vi "getXMLCameraPlacement.vi"(9 "usb/watec":bool, 11 "path to XML document":path=path "C:/BeamPointing/trunk/Beam Pointing v22 Library/xml Settings/ConfigFile.xml") -> (0 "error out":errorcluster, 1 "parse errors":string, 2 "Default devices":string[](array[string]), 3 "Cameras names/#":T1(array[cluster]), 5 "Default Cameras Names":string[](array[string]))   [LabVIEW 2013]
uses:
  <vilib>/xml/Load XML File.vi
  <vilib>/xml/NI_XML.lvlib
  <resource>/objmgr/DOMUserDefRef.rc
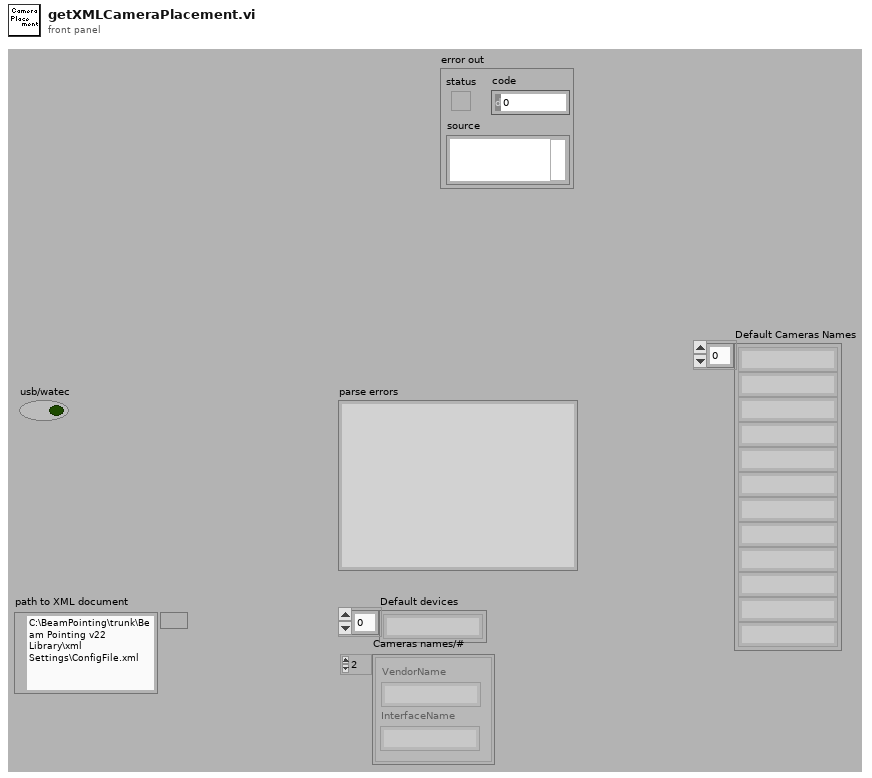
[diagram p1: front panel]
types:
  T1 = cluster{"VendorName":string, "InterfaceName":string}[]
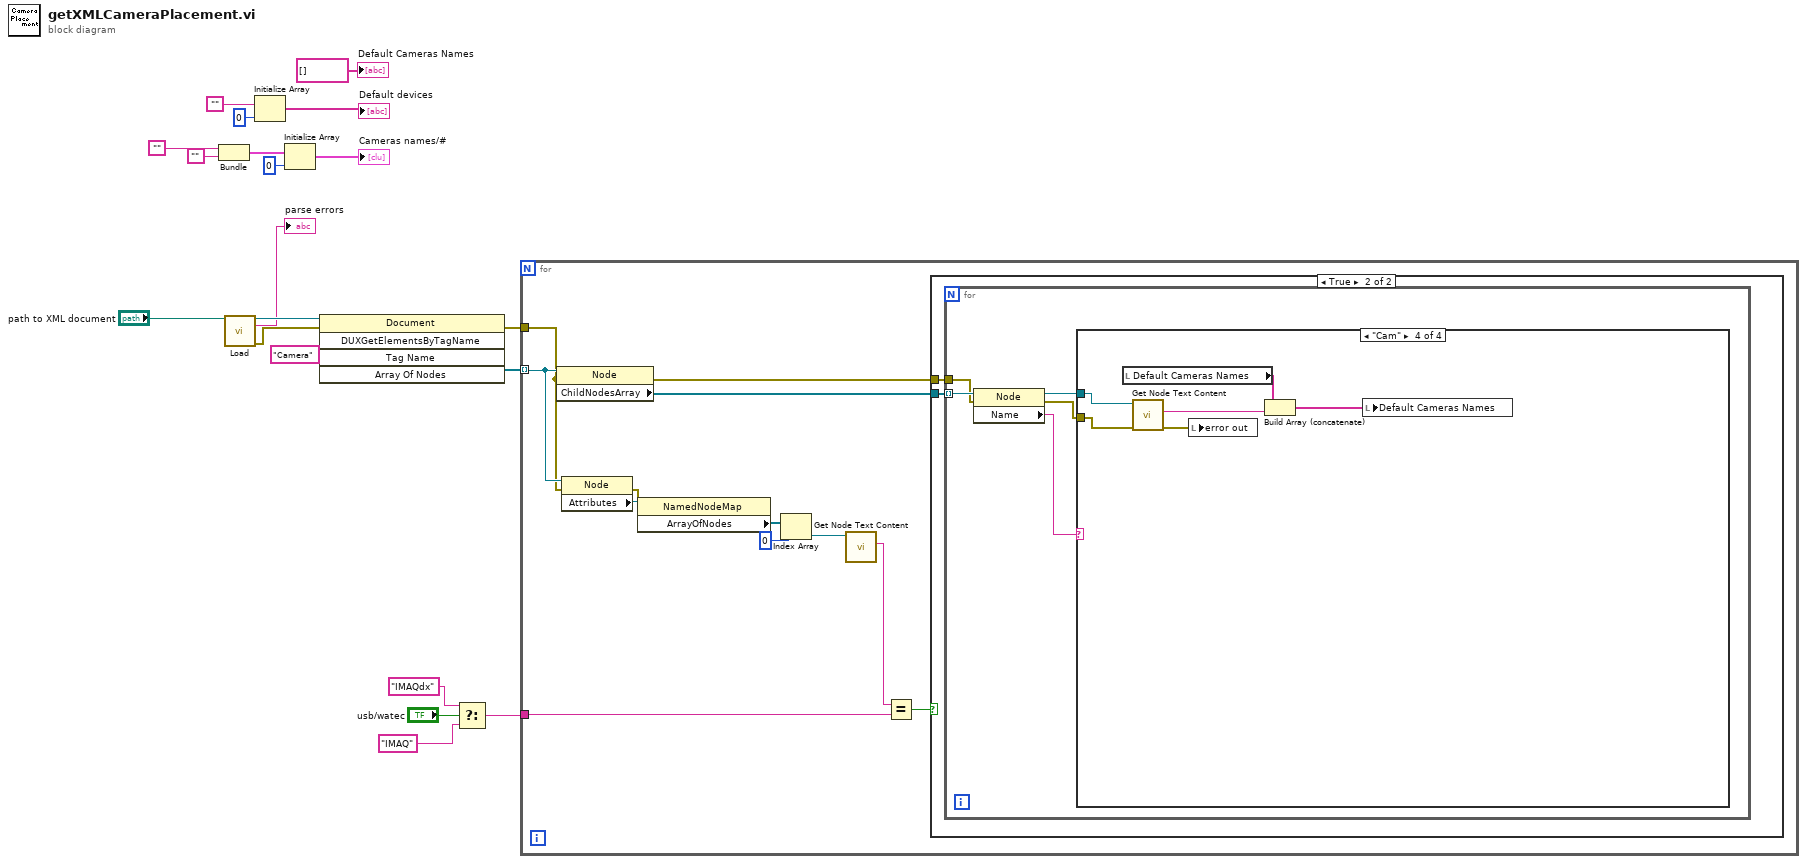
[diagram p0: block diagram]
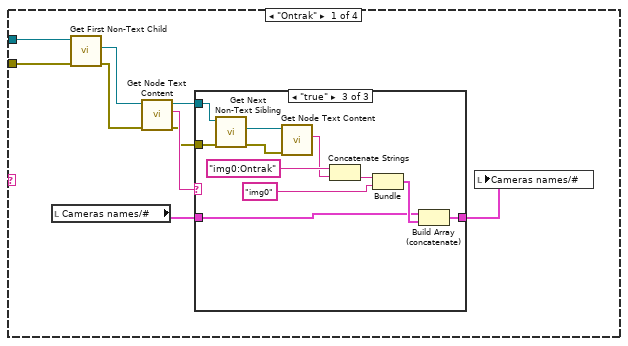
[diagram p3: hidden frame]
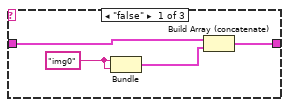
[diagram p4: hidden frame]
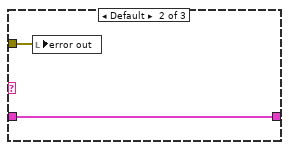
[diagram p5: hidden frame]
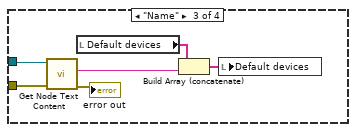
[diagram p7: hidden frame]
diagram:
  n1 = Bundle("", "") -> (w8:cluster{string, string})  [unwired: 1 in]
  n2 = call-poly <vilib>:"Load.vi"("path to XML document"="path to XML document") -> ("DOM document out"=w19:refnum<k20>, "parse errors"=→"parse errors":string, "error out"=w18:errorcluster)  [unwired: 12 in]
  n3 = Initialize Array("", 0 ("dimension size")) -> (→"Default devices":string[])
  n4 = Initialize Array(w8, 0 ("dimension size")) -> (→"Cameras names/#":cluster{string, string}[])
  n5 = invoke class="Document" method="DUXGetElementsByTagName"(reference=w19, error in=w18, "Tag Name"="Camera") -> (error out=w5:errorcluster, "Array Of Nodes"=w17:refnum<k20>[])  [unwired: 2 in, 3 out]
  n6 = Select(t="IMAQdx", s="usb/watec", f="IMAQ") -> (s? t:f=w2:string)
  n7 = for {
    tunnel: w17 -> [w31] mode=indexing
    tunnel: w5 -> [w29]
    tunnel: w2 -> [w23]
    n8 = property class="Node"(reference=w31, error in=w29) -> (error out=w21:errorcluster, "ChildNodesArray"=w32:refnum<k20>[])  [unwired: 1 out]
    n9 = property class="Node"(reference=w31, error in=w29) -> (error out=w28:errorcluster, "Attributes"=w30:refnum<k20>)  [unwired: 1 out]
    n10 = property class="NamedNodeMap"(reference=w30, error in=w28) -> ("ArrayOfNodes"=w27:refnum<k20>[])  [unwired: 2 out]
    n11 = Index Array(array=w27, index=0) -> (element=w25:refnum<k20>)
    n12 = call <vilib>:"Get Node Text Content.vi"("node in"=w25) -> ("node text"=w24:string)  [unwired: 8 in, 2 out]
    n13 = Equal?(x=w24, y=w23) -> (x = y?=w22:bool)
    n14 = case shown="True" w22 {
      tunnel: w32 -> [_ w34]
      tunnel: w21 -> [_ w33]
      frame False {
      }
      frame True {
        n15 = for {
          tunnel: w34 -> [w39] mode=indexing
          tunnel: w33 -> [w36]
          n16 = property class="Node"(reference=w39, error in=w36) -> (reference out=w37:refnum<k20>, error out=w35:errorcluster, "Name"=w38:string)
          n17 = case shown="\"Cam\"" w38 {
            tunnel: w37 -> [w48 _ w71 w73]
            tunnel: w35 -> [w41 _ w67 w72]
            frame "Ontrak" {
              n18 = local read "Cameras names/#"() -> (w45:T1)
              n19 = call <vilib>:"Get First Non-Text Child.vi"("error in (no error)"=w41, "node in"=w48) -> ("error out"=w47:errorcluster, "child node"=w43:refnum<k20>)  [unwired: 6 in, 2 out]
              n20 = call <vilib>:"Get Node Text Content.vi"("error in (no error)"=w47, "node in"=w43) -> ("error out"=w40:errorcluster, "node text"=w46:string, "node out"=w42:refnum<k20>)  [unwired: 7 in]
              n21 = case shown="\"true\"" w46 {
                tunnel: w45 -> [w51 w54 w61]
                tunnel: [w49 w54 w60] -> w44
                tunnel: w42 -> [_ _ w56]
                tunnel: w40 -> [_ w53 w55]
                frame "false" {
                  w52 = "img0"
                  n22 = Bundle(w52, w52) -> (w50:cluster{string, string})  [unwired: 1 in]
                  n23 = Build Array (concatenate)(w51, w50) -> (w49:T1)
                }
                frame Default {
                  n24 = local write "error out"(w53) -> ()
                }
                frame "true" {
                  n25 = call <vilib>:"Get Next Non-Text Sibling.vi"("error in (no error)"=w55, "node in"=w56) -> ("error out"=w58:errorcluster, "sibling node"=w59:refnum<k20>)  [unwired: 6 in, 2 out]
                  n26 = call <vilib>:"Get Node Text Content.vi"("error in (no error)"=w58, "node in"=w59) -> ("node text"=w57:string)  [unwired: 7 in, 2 out]
                  n27 = Concatenate Strings("img0:Ontrak" ("string"), w57) -> (w64:string)
                  n28 = Bundle(w64, "string"="img0") -> (w62:cluster{string, "string":string})  [unwired: 1 in]
                  n29 = Build Array (concatenate)(w61, w62) -> (w60:cluster{"VendorName":string, "string":string}[])
                }
              }
              n30 = local write "Cameras names/#"(w44) -> ()
            }
            frame Default {
            }
            frame "Name" {
              n31 = call <vilib>:"Get Node Text Content.vi"("error in (no error)"=w67, "node in"=w71) -> ("error out"=→"error out":errorcluster, "node text"=w69:string)  [unwired: 7 in, 1 out]
              n32 = local read "Default devices"() -> (w70:string[])
              n33 = Build Array (concatenate)(w70, w69) -> (w68:string[])
              n34 = local write "Default devices"(w68) -> ()
            }
            frame "Cam" {
              n35 = local read "Default Cameras Names"() -> (w76:string[])
              n36 = call <vilib>:"Get Node Text Content.vi"("error in (no error)"=w72, "node in"=w73) -> ("error out"=w77:errorcluster, "node text"=w75:string)  [unwired: 7 in, 1 out]
              n37 = local write "error out"(w77) -> ()
              n38 = Build Array (concatenate)(w76, w75) -> (w74:string[])
              n39 = local write "Default Cameras Names"(w74) -> ()
            }
          }
        }
      }
    }
  }
  "Default Cameras Names" <- string[] [] ("Cameras Names")
